vi "Run all tests.vi"() -> ()   [LabVIEW 2020]
uses:
  <vilib>/addons/_JKI Toolkits/Caraya/classes/Test Result/Test Result.lvclass
  <vilib>/addons/_JKI Toolkits/Caraya/classes/Test Report/Test Report.lvclass
  <vilib>/addons/_JKI Toolkits/Caraya/Caraya.lvlib
  <vilib>/addons/_JKI Toolkits/Caraya/run-tests/Run Test (Scalar Path).vi
panel:
  in  "Test Report":refnum<class "Test Report.lvclass">
  out "Test Results":refnum<class "Test Result.lvclass">
  out "error out":errorcluster
  in  "Interactive (T)":bool=TRUE
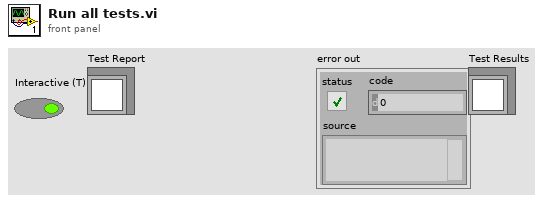
[diagram p1: front panel]
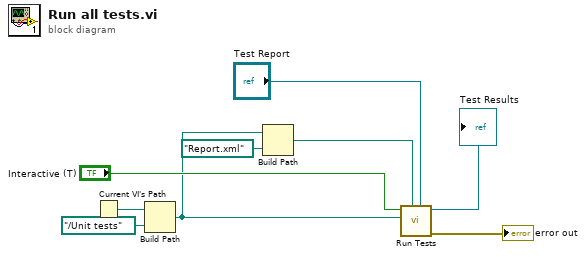
[diagram p0: block diagram]
diagram:
  n1 = Current VI's Path() -> (path=w9:path)
  n2 = Build Path(base path=w9, name or relative path=path "../Unit tests") -> (appended path=w3:path)
  n3 = Build Path(base path=w3, name or relative path=path "Report.xml") -> (appended path=w1:path)
  n4 = call-poly <vilib>:"Run Tests.vi"("Test Report"="Test Report", "Report Path"=w1, "Test Path"=w3, "Interactive (T)"="Interactive (T)") -> ("error out"=→"error out":errorcluster, "Test Results"=→"Test Results":refnum<class "Test Result.lvclass">)  [unwired: 6 in]
